vi "Img Update Frame Image.vi"(8 "error in (no error)":errorcluster, 11 "LF2R IDE in":refnum<class "Main Panel.lvclass">) -> (0 "error out":errorcluster, 3 "LF2R IDE out":refnum<class "Main Panel.lvclass">)   [LabVIEW 2018, in "Main Panel.lvlib" / "Main Panel.lvclass"]
uses:
  Main Panel.lvclass
  Main Panel.lvclass/Main Panel.ctl
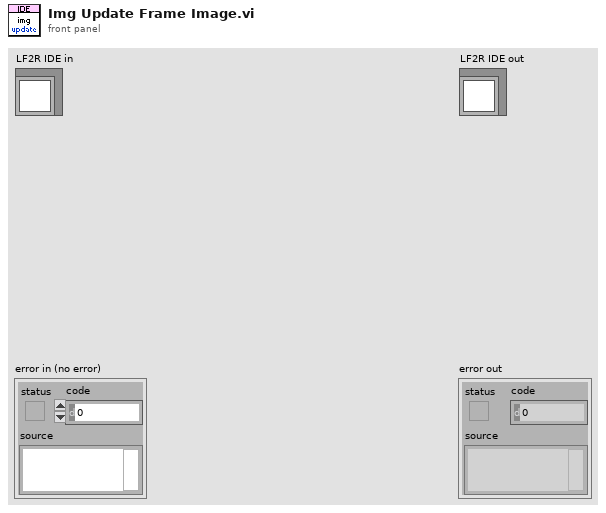
[diagram p1: front panel]
types:
  T1 = typedef "imagedata.ctl" = cluster{"image type":i32, "image depth":i32, "image":u8[], "mask":u8[], "colors":u32[], "Rectangle":cluster{"left":i16, "top":i16, "right":i16, "bottom":i16}}
  T2 = typedef "Image Json Parser.lvclass/Img Json Data.ctl" = cluster{"frames":T3[], "meta":T4}
  T3 = typedef "Image Json Parser.lvclass/Img Json Frames.ctl" = cluster{"frame":cluster{"x":i32, "y":i32, "w":i32, "h":i32}, "rotated":bool, "trimmed":bool, "spriteSourceSize":cluster{"x":i32, "y":i32, "w":i32, "h":i32}, "sourceSize":cluster{"w":i32, "h":i32}}
  T4 = typedef "Image Json Parser.lvclass/Img Json Meta.ctl" = cluster{"app":string, "version":string, "image":string, "format":string, "size":cluster{"w":i32, "h":i32}, "scale":string}
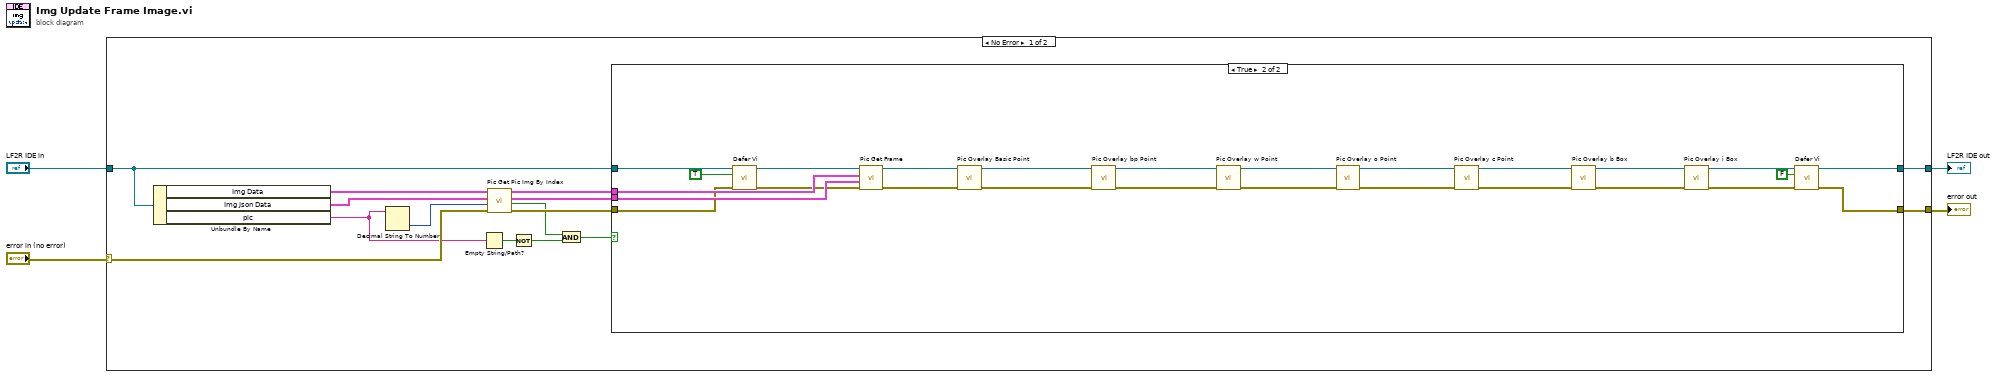
[diagram p0: block diagram]
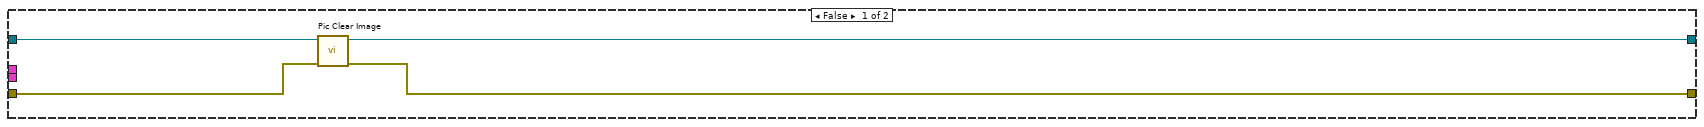
[diagram p2: hidden frame]
diagram:
  n1 = case shown="No Error" "error in (no error)" {
    selector: "error in (no error)" -> [w17 w51]
    tunnel: [w13 w51] -> w3
    tunnel: [w5 w50] -> w1
    tunnel: "LF2R IDE in" -> [w6 w50]
    frame No Error {
      n2 = Unbundle By Name(w6) -> ("Img Data"=w19:cluster{"image data":T1, "bitmap":u32[][]}[], "Img Json Data"=w18:T2[], "pic"=w11:string)
      n3 = Decimal String To Number(string=w11) -> (number=w12:i32)  [unwired: 2 in, 1 out]
      n4 = Empty String/Path?(string/path=w11) -> (empty?=w10:bool)
      n5 = call "Pic Get Pic Img By Index.vi"("error in (no error)"=w17, "Pic Num"=w12, "Img Json Data"=w18, "Img Data"=w19) -> ("error out"=w14:errorcluster, "Found?"=w8:bool, "frames"=w16:T3, "Img Data Indexed"=w15:cluster{"image data":T1, "bitmap":u32[][]})  [unwired: 4 in]
      n6 = Not(x=w10) -> (.not. x?=w9:bool)
      n7 = And(x=w8, y=w9) -> (x .and. y?=w7:bool)
      n8 = case shown="True" w7 {
        tunnel: w16 -> [_ w48]
        tunnel: w15 -> [_ w49]
        tunnel: w14 -> [w22 w28]
        tunnel: [w21 w24] -> w13
        tunnel: w6 -> [w23 w29]
        tunnel: [w20 w25] -> w5
        frame False {
          n9 = call "Pic Clear Image.vi"("error in (no error)"=w22, "LF2R IDE in"=w23) -> ("error out"=w21:errorcluster, "LF2R IDE out"=w20:refnum<class "Main Panel.lvclass">)  [unwired: 8 in]
        }
        frame True {
          n10 = call "Defer Vi.vi"("error in (no error)"=w28, "Defer Updates?"=TRUE, "Main Panel in"=w29) -> ("error out"=w32:errorcluster, "Main Panel out"=w33:refnum<class "Main Panel.lvclass">)  [unwired: 7 in]
          n11 = call "Pic Get Frame.vi"("error in (no error)"=w32, "frames"=w48, "Img Data indexed"=w49, "LF2R IDE in"=w33) -> ("error out"=w46:errorcluster, "LF2R IDE out"=w47:refnum<class "Main Panel.lvclass">)  [unwired: 6 in]
          n12 = call "Pic Overlay Basic Point.vi"("error in (no error)"=w46, "LF2R IDE in"=w47) -> ("error out"=w44:errorcluster, "LF2R IDE out"=w45:refnum<class "Main Panel.lvclass">)  [unwired: 8 in]
          n13 = call "Pic Overlay bp Point.vi"("error in (no error)"=w44, "LF2R IDE in"=w45) -> ("error out"=w42:errorcluster, "LF2R IDE out"=w43:refnum<class "Main Panel.lvclass">)  [unwired: 8 in]
          n14 = call "Pic Overlay w Point.vi"("error in (no error)"=w42, "LF2R IDE in"=w43) -> ("error out"=w40:errorcluster, "LF2R IDE out"=w41:refnum<class "Main Panel.lvclass">)  [unwired: 8 in]
          n15 = call "Pic Overlay o Point.vi"("error in (no error)"=w40, "LF2R IDE in"=w41) -> ("error out"=w38:errorcluster, "LF2R IDE out"=w39:refnum<class "Main Panel.lvclass">)  [unwired: 8 in]
          n16 = call "Pic Overlay c Point.vi"("error in (no error)"=w38, "LF2R IDE in"=w39) -> ("error out"=w36:errorcluster, "LF2R IDE out"=w37:refnum<class "Main Panel.lvclass">)  [unwired: 8 in]
          n17 = call "Pic Overlay b Box.vi"("error in (no error)"=w36, "LF2R IDE in"=w37) -> ("error out"=w34:errorcluster, "LF2R IDE out"=w35:refnum<class "Main Panel.lvclass">)  [unwired: 8 in]
          n18 = call "Pic Overlay i Box.vi"("error in (no error)"=w34, "LF2R IDE in"=w35) -> ("error out"=w30:errorcluster, "LF2R IDE out"=w31:refnum<class "Main Panel.lvclass">)  [unwired: 8 in]
          n19 = call "Defer Vi.vi"("error in (no error)"=w30, "Defer Updates?"=FALSE, "Main Panel in"=w31) -> ("error out"=w24:errorcluster, "Main Panel out"=w25:refnum<class "Main Panel.lvclass">)  [unwired: 7 in]
        }
      }
    }
    frame Error {
    }
  }
  "error out" <- w3
  "LF2R IDE out" <- w1
